vi "数据处理.vi"(6 "原始数据文件名":string="AI0.csv", 7 "去噪信号保存的文件名":string="AI100.csv", 9 "数组中的数据（输入）":dbl[](array[numeric]), 10 "小波包变换":refnum<k7>, 11 "信号去燥":refnum<k7>) -> (1 "字符串（输出）":string, 2 "特征值（输出）":dbl[][](array[numeric]), 3 "去噪后波形图":dbl[][](graph))   [LabVIEW 2018]
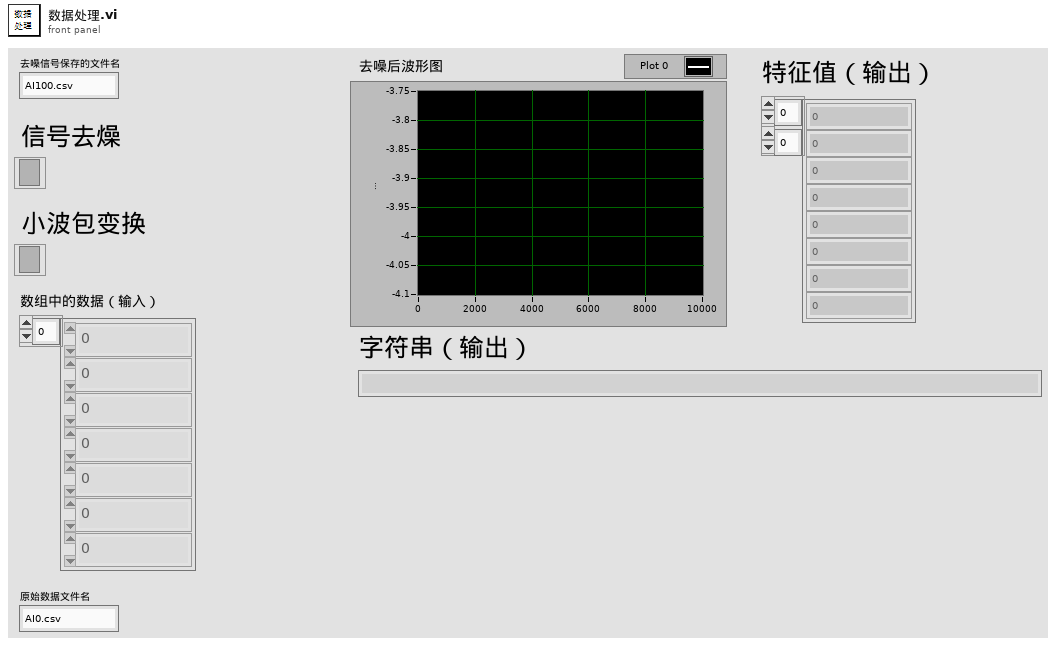
[diagram p1: front panel]
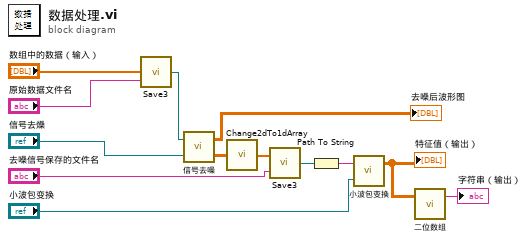
[diagram p0: block diagram]
diagram:
  n1 = call "Save3.vi"("要保存的文件名（输入）"="原始数据文件名", "数组中的数据（输入）"="数组中的数据（输入）") -> ("文件保存路径（输出）"=w9:path)
  n2 = call "信号去噪.vi"("Automation Refnum in"="信号去燥", "文件路径（输入）"=w9) -> ("去噪后数据输出"=w5:dbl[][], "去噪后波形图（输出）"=→"去噪后波形图":dbl[][])
  n3 = call "Change2dTo1dArray.vi"("AI2去噪后数据"=w5) -> ("AI2一维数组"=w4:dbl[])
  n4 = call "Save3.vi"("要保存的文件名（输入）"="去噪信号保存的文件名", "数组中的数据（输入）"=w4) -> ("文件保存路径（输出）"=w7:path)
  n5 = Path To String(path=w7) -> (string=w6:string)
  n6 = call "小波包变换.vi"("Automation Refnum in"="小波包变换", "数据文件路径（输入）"=w6) -> ("特征值（输出）"=w2:dbl[][])  [unwired: 1 in]
  "特征值（输出）" <- w2
  n7 = call "二位数组.vi"("二位数组（输入）"=w2) -> ("字符串（输出）"=→"字符串（输出）":string)  [unwired: 1 in, 1 out]
